vi "toggle listbox checks.vi"(8 "error in (no error)":errorcluster, 11 "ListBox in":refnum<vi>) -> (0 "error out":errorcluster, 2 "selected values":bool[](array[boolean]))   [LabVIEW 2016, in "FPGA RM System Definition API.lvlib"]
uses:
  FPGA RM System Definition API.lvlib
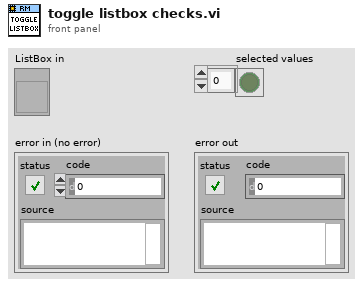
[diagram p1: front panel]
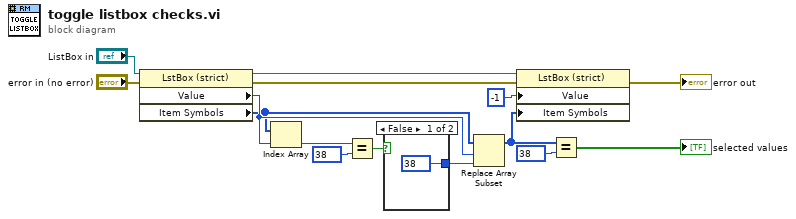
[diagram p0: block diagram]
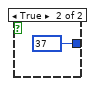
[diagram p2: hidden frame]
diagram:
  n1 = property class="LstBox (strict)"(reference="ListBox in", error in="error in (no error)") -> (reference out=w11:refnum<vi>, error out=w14:errorcluster, "Value"=w10:i32, "Item Symbols"=w9:i32[])
  n2 = Index Array(array=w9, index=w10) -> (element=w7:i32)
  n3 = Equal?(x=w7, y=38) -> (x = y?=w6:bool)
  n4 = case shown="False" w6 {
    tunnel: [38 37] -> w12
    frame False {
    }
    frame True {
    }
  }
  n5 = Replace Array Subset(array=w9, new element=w12, index=w10) -> (w3:i32[])
  n6 = property class="LstBox (strict)"(reference=w11, error in=w14, "Value"=-1, "Item Symbols"=w3) -> (error out=→"error out":errorcluster)  [unwired: 1 out]
  n7 = Equal?(x=w3, y=38) -> (x = y?=→"selected values":bool[])
